vi "AlliGator All ROIs IRF Analysis.vi"(8 "error in (no error)":errorcluster, 11 "AlliGator Internal Variables DVR":refnum<data-value>) -> (0 "error out":errorcluster, 1 "# IRFs defined":i32, 2 "Message":string, 3 "AlliGator Internal Variables DVR":refnum<data-value>)   [LabVIEW 2021, in "AlliGator IRF.lvlib"]
doc: "Extracts the decays from all ROIs and stores them as IRFs for subsequent NLSF analysis."
uses:
  AlliGator IRF.lvlib
  Internal Variables/AlliGator Internal Variables v2.ctl
  <vilib>/vision/Image Controls.llb/IMAQ Image.ctl
  Internal Variables/AlliGator Gate Image Set.ctl
  Files/AlliGator FLI Dataset Type.ctl
  Files/AlliGator Data Series Type.ctl
  Dual-Channel Datasets/AlliGator Dataset Channel.ctl
  Settings/AlliGator Gate Arithmetic.ctl
  Source Image/AlliGator Displayed Image.ctl
  Image/Named ROI Description.ctl
  Phasor Graph/AlliGator Decay Metadata v3.ctl
  Decay Preprocessing/AlliGator Decay Background Subtraction Info.ctl
  Decay Preprocessing/AlliGator Baseline Subtraction Method.ctl
  Graphs/XY Graph/XY Graph Plot Shift Parameters.ctl
  Graphs/XY Graph/XY Graph Plot Shift Method.ctl
  Decay Preprocessing/AlliGator Decay Extrapolation Parameters.ctl
  Phasor/Calibration Phasor (m, phi).ctl
  Phasor/Phasor Reference Series.ctl
  Phasor/Phasor Calibration Map v2.ctl
  Phasor/Phasor (g, s).ctl
  Phasor Graph/AlliGator Raw Phasor Plot Data v5.ctl
  Phasor/Phasor Standard Deviation Options.ctl
  Phasor Plot/AlliGator Phasor Multi-Harmonic Data.ctl
  Phasor/Phasor Harmonic Data.ctl
  Decay Fit Parameter Map/AlliGator Decay Fit Options & Parameters v4.ctl
  Fits/IRF(X)PSED/Decay Fit Options v4.ctl
  Fits/Decay Convolution/Decay Model.ctl
  Fits/Residual Type.ctl
  Fits/IRF(X)PSED/Fit Weights Type v2.ctl
  Fits/Non-linear Fitting Method v2.ctl
  Fits/Fit Calculation Method.ctl
  Fits/Non-linear Fitting Algorithm.ctl
  Decay Fit/AlliGator Decay Fit Parameter Constraints 2.ctl
  Fits/IRF(X)PSED/Decay Fit Parameters In List.ctl
  Fits/IRF(X)PSED/MLE Baseline Offset Type.ctl
  Decay Preprocessing/AlliGator Decay Preprocessing Parameters.ctl
  Fits/IRF(X)PSED/Decay Fit Parameters & Derived Quantities List v2.ctl
  Fits/IRF(X)PSED/Decay Fit Result Constraint.ctl
  Decay Fit Parameter Map/AlliGator Parameter Maps Data.ctl
  Globals, Variables, Constants/AlliGator Variables List.ctl
  Rich Text Box/Text Format List.ctl
  Variant/Variant to Data/Variant to U16.vi
  <vilib>/Utility/error.llb/Error Cluster From Error Code.vi
  Globals, Variables, Constants/AlliGator Abort.vi
  <vilib>/ErrorRing/Error Ring.xnode
  Globals, Variables, Constants/AlliGator Globals, Variables & Constants.lvlib
  Image/Image.lvlib
  Decay Processing/AlliGator Decay Processing.lvlib
  Source Image/AlliGator Source Image.lvlib
  Strings/Strings.lvlib
  Time/Time.lvlib
  Decay Preprocessing/AlliGator Decay Preprocessing.lvlib
  Notebook/Notebook.lvlib
  GUI/GUI.lvlib
  Variant/Variant to Data/Variant to Data.lvlib
  Utilities/Utilities.lvlib
  Phasor/Phasor.lvlib
  Files/AlliGator Files.lvlib
  Internal Variables/AlliGator Internal Variables.lvlib
  Phasor Graph/AlliGator Phasor Graph.lvlib
  Graphs/XY Graph/XY Graph Add-Ons.lvlib
  Phasor Plot/AlliGator Phasor Plot.lvlib
  Fits/Fits.lvlib
  Decay Fit/AlliGator Decay Fit.lvlib
  Settings/AlliGator Settings.lvlib
  Dual-Channel Datasets/AlliGator Dual-Channel Datasets.lvlib
  Decay Fit Parameter Map/AlliGator Decay Fit Parameter Map.lvlib
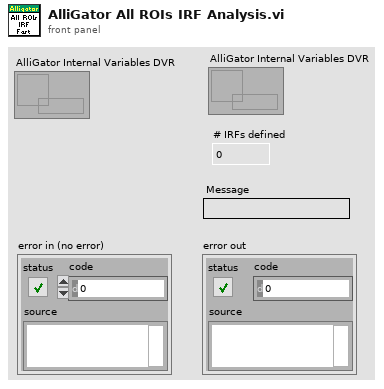
[diagram p1: front panel]
types:
  T1 = typedef "AlliGator Globals, Variables & Constants.lvlib/AlliGator Variables List.ctl" = enum16{"---- GUI ----", "GUI:Initialization Status", "GUI:State Indicators Refnum", "GUI:Original AlliGator Menu Items", "GUI:Current Action Loop State", "GUI:Script in progress", "GUI:Playback", "GUI:Loop Playback", "GUI:Search ROI Used", "GUI:Search ROI", "Decay Graph Max Legend Size", "Intensity Graph Max Legend Size", "Decay Statistics Graph Max Legend Size", "Phasor Graph Max Legend Size", "Phasor Ratio Graph Max Legend Size", "Lifetime Graph Max Legend Size", "---- Files ----", "Files:Export Dataset Frames as Individual Files", "Files:Show Batch Export Help Balloons", "Files:Frames in Dataset", "Files:ptu File Frame Start Indices", "Files:Current Frame in Dataset", "Files:Current Frame Timestamp", "Files:Dataset Loaded", "Files:Dataset Metadata", "Files:Dataset Channel", "Files:Dataset Data Description", "Files:Background Dataset Metadata", "Files:Background Dataset Channel", "Files:Background Dataset Data Description", "Files:Background File Subtraction", "Files:Background File Path", "Files:Background File Pile-up Correction", "Files:Background File Pixel Well Capacity", "Files:Background File Scaling Factor", "Files:Current Dataset Load Settings", "Files:Dataset Path", "Files:ICCD-specific Information", "Files:Macrotime Gate Separation", "------ Python Plugins ------", "Python Plugins:Information", "Python Plugins:Python Session", "Python Plugins:Valid Python Session?", "---- Source Image ----", "Source Image:ROIs", "Source Image:Current ROI", "Source Image:ROI Event Refnum", "X_Source Image:Display Range", "X_Source Image:Palette Information", "X_Source Image:Type of Displayed Image", "X_Time Gate Slider", "Source Image:Palette List", "Source Image:Scale", "Source Image:ROI Overlay Color", "Source Image:Overlay to Erase", "Source Image:Is Displayed Image Accumulated", "Source Image:White Light Image Modified", "Source Image:Mask Image Modified", "---- Image Profile Window ----", "Image Profile:Window Event Refnum", "Image Profile:IntensityType", "Image Profile:Intensity Average Type", "Image Profile:Intensity-weighted SDV", "Image Profile:Box Profile Type", "Image Profile:Window Open", "Image Profile:Plotted Fit Parameter", "------ Phasor Graph -------", "Phasor Graph:Show Line", "---- Phasor Plot ---", "Phasor Plot:Parameters Changed", "Phasor Plot:FLI Dataset Modified since last Calculation", "Phasor Harmonics Data", "Selected Phasor Harmonics", "Phasor Harmonic Manager Event Refnum", "Phasor Plot:ROIs", "Phasor Plot:Current ROI", "Phasor Plot:ROI Event Refnum", "Phasor Plot:Image Reference Points", "Phasor Plot:Computed", "Phasor Plot:Palette Information", "Phasor Plot:Palette List", "Phasor Plot:Phasor Ratio Palette Information", "Phasor Plot:Phasor Ratio Palette List", "Phasor Plot:Image Scale", "Phasor Plot:Image Overlay to Erase", "Phasor Plot:Image Elements to Update", "Phasor Plot:Current Calculation Parameters", "Phasor Plot:Current Calibration Options", "Phasor Plot:Reset Cumulated Phasor Plot", "Phasor Plot:Reference 1", "Phasor Plot:Lifetime Reference 1", "Phasor Plot:Reference 1 Frequency", "Phasor Plot:Reference 2", "Phasor Plot:Lifetime Reference 2", "Phasor Plot:Reference 2 Frequency", "---- Decay Analysis ----", "Number of Selected Decays to Fit", "LS Fit Results", "LAR Fit Results", "BS Fit Results", "Last Decay Max - Min", "Best Fit Parameters", "Best Fit Parameter Names", "Actual Size X", "Actual Size Y", "Binning X", "Binning Y", "Actual # Gates", "Dataset Number", "Gates to...", "Gates Skipped", "Gates to keep", "Gate Step", "Gate Separation", "Reversed Gates", "Pile-up Correction", "Pixel Well Capacity", "Background Subtracted", "Background Subtraction Method", "Background Definition Range", "Background File (deprecated)", "Number of Dataset Accumulated", "Array of Accumulated Dataset Paths", "Do Averaged Datasets", "Destination File Path", "Process Plot Target", "Use 1/D as Phasor Frequency", "---- Decay Fit Parameter Map -----", "Decay Fit Parameter Map:Palette Information", "Decay Fit Parameter Map:Palette List", "Decay Fit Parameter Map:X Resolution", "Decay Fit Parameter Map:Y Resolution", "Decay Fit Parameter Map:Use Decay Fit Result Constraints", "Decay Fit Parameter Map:Decay Fit Result Constraints", "Decay Fit Parameter Map:Decay Fit Result Constraints Applied", "---- Parameter Map ----", "Parameter Map:Palette Information", "Parameter Map:Palette List", "------- Local Decay Window ---------", "Local Decay Graph Window:Event Refnum", "Local Decay Graph Window:Use normalized IRF for convolution", "----- Miscellaneous ----", "Misc:Skippable Dialog Windows Status"}
  T2 = typedef "IMAQ Image.ctl" = refnum<image>
  T3 = typedef "Image.lvlib/Named ROI Description.ctl" = cluster{"ROI Descriptor":T4, "ROI Name":string, "Overlay Color":u32}
  T4 = typedef "ROI Descriptor" = cluster{"Global Rectangle":i32[], "Contours":cluster{"ID":enum32{"External", "Internal"}, "Type":u32, "Coordinates":i32[]}[]}
  T5 = typedef "Notebook.lvlib/Text Format List.ctl" = enum16{"Message", "Result", "Error", "Setting", "Verbose", "Warning"}
  T6 = typedef "AlliGator Internal Variables.lvlib/AlliGator Internal Variables v2.ctl" = cluster{"----------------------------- Images -----------------------------":u8, "Displayed Image":T2, "White Light Image":T2, "Mask Image":T2, "ROI Mask Image":T2, "Current Dataset Images 1":T7, "Background Dataset Images 1":T7, "Current Dataset Images 2":T7, "Background Dataset Images 2":T7, "Current Dataset Arithmetic Images":T7, "Accumulated Dataset Images 1":T7, "Accumulated Dataset Images 2":T7, "Accumulated Dataset Arithmetic Images":T7, "----------------------------- File Paths -----------------------------":u8, "Phasor Plot Image":T2, "Decay Fit Parameter Map Image":T2, "Parameter Map Image":T2, "Single Data Point Path":path, "White Light Image Path":path, "Mask Image Path":path, "Time-Series Folder":path, "[Time-Series Paths]":path[], "----------------------------- FLI Dataset -----------------------------":u8, "Current Dataset":i32, "Single Dataset Type":T8, "Current Folder":string, "AlliGator Data Series Type":T9, "# Datasets":i32, "Dual-Channel Dataset":bool, "Selected Channel Name":string, "Dataset Channel":T10, "Channel Arithmetic":T11, "Dual-Channel Background Dataset":bool, "Background Channel":T10, "Dual-Channel Accumulated Dataset":bool, "Start Time":dbl, "[Time-Series Timestamps]":dbl[], "[Intensity Corrections]":dbl[], "Time Series Script":bool, "Type of Displayed Image":T12, "Gate Image Slide":u16, "# Gates":i32, "ROIs":T3[], "----------------------------- Decays -----------------------------":u8, "ROI Decay":cluster{"t Array":dbl[], "I Array":dbl[]}, "Valid Decay":bool, "Decay  Metadata":T13, "Reference Decay Plot Name":string, "Reference Decay":cluster{"t Array":dbl[], "I Array":dbl[]}, "Decay Shift Plot":cluster{"Time Stamps":dbl[], "Decay Shifts":dbl[]}, "[Decays Max Values]":sgl[], "[Decays Min Values]":sgl[], "----------------------------- Calibration -----------------------------":u8, "Calibration Phasor":T19, "Calibration Phasor Series":T20, "Phasor Calibration Map":T21, "Calibration Map MD5 Digest":string, "----------------------------- Phasor Graph -----------------------------":u8, "Last Raw Phasor":T22, "Last Calibrated Phasor":T22, "Last Calibrated Phasor SDV":T22, "Phasor Graph:Phasor Plot":cluster{"g Array":dbl[], "s Array":dbl[]}, "Phasor Graph:Phasor SDV Plot":cluster{"g Array":dbl[], "s Array":dbl[]}, "[Phasor Graph:Raw Phasor Plots]":T23[], "Phasor Plot locked to Ref 1":i32, "[Phasor Plot(s) locked to Ref 1]":i32[], "[Phasor Plot(s) locked to Ref 2]":i32[], "[Pixel Phasors]":T22[], "----------------------------- Phasor Plot -----------------------------":u8, "[[Sum Image]]":dbl[][], "[[CSG Phasors]]":csg[][], "[[Valid Pixel?]]":bool[][], "[[Phasor Ratios]]":dbl[][], "[[Average Lifetimes]]":dbl[][], "Amplitude Weighted Average Lifetime":bool, "I/m/phi Dataset":cluster{"I/m/phi Dataset?":bool, "Base Frequency":dbl[unit], "Harmonic Orders":u8[]}, "Multi Phasor Plot Data":T25, "----------------------------- Decay Fit Parameter Map -----------------------------":u8, "Decay Fit Options & Parameters":T27, "Fit Options: Decay Preprocessing Parameters":T38, "Fit Options: Reference Decay":cluster{"t Array":dbl[], "I Array":dbl[]}, "Is Full Image Parameters Map":bool, "Is Single-Pixels Parameters Map":bool, "NLSF Parameters Map X Resolution":i32, "NLSF Parameters Map Y Resolution":i32, "[Single Decay Fit Parameters]":dbl[], "Fit Model":T29, "[[Multiple Decays Fit Parameters]]":dbl[][], "[[Multiple Decays Fit Parameter SDVs]]":dbl[][], "[[IRFs]]":dbl[][], "[ROI Descriptors]":T4[], "IRF Array Time Axis":dbl[], "Decay Array Time Axis":dbl[], "[Decay Fit Parameter Names]":T39[], "[Decay Sum]":dbl[], "Array of Decay Fit Result Constraints":T40[], "Selected ROIs Array":bool[], "----------------------------- Parameter Maps -----------------------------":u8, "[Map Set Names]":string[], "[Parameter Maps]":T41[], "[[User-defined Quantities]]":dbl[][], "User-defined Quantity":string}
  T7 = typedef "AlliGator Internal Variables.lvlib/AlliGator Gate Image Set.ctl" = cluster{"SGL Gate Images":T2[], "SGL Sum Image":T2, "SGL Max Image":T2, "SGL Min Image":T2}
  T8 = typedef "AlliGator Files.lvlib/AlliGator FLI Dataset Type.ctl" = enum16{"HDF5 FLI Dataset", "Gate Image Folder", ".sdt FLI Dataset (Becker & Hickl)", ".ptu FLI Dataset (PicoQuant)", "SS1 FLI Dataset", "SS2 FLI Dataset", "I/m/phi Dataset", ".bin FLI Dataset (PicoQuant Binned)", ".bin FLI Dataset (Piccolo Binned)", ".mat FLI Dataset"}
  T9 = typedef "AlliGator Files.lvlib/AlliGator Data Series Type.ctl" = enum16{"Not a Supported Series", "Gate Images Folder Series", "SwissSPAD 2 Dataset Series", "B&H FLI Dataset Series", "PicoQuant PTU FLI Dataset Series", "PicoQuant BIN FLI Dataset Series", "Piccolo hist BIN FLI Dataset Series", "HDF5 FLI Dataset Series"}
  T10 = typedef "AlliGator Dual-Channel Datasets.lvlib/AlliGator Dataset Channel.ctl" = enum16{"G2", "INT"}
  T11 = typedef "AlliGator Settings.lvlib/AlliGator Gate Arithmetic.ctl" = enum16{"None", "INT-G2", "G2/INT*<INT>", "(1 - G2/INT)*<INT>"}
  T12 = typedef "AlliGator Source Image.lvlib/AlliGator Displayed Image.ctl" = enum16{"Single Gate", "Sum of All Gates", "Max of All Gates", "Min of All Gates", "-", "White Ligth Image", "Mask Image"}
  T13 = typedef "AlliGator Phasor Graph.lvlib/AlliGator Decay Metadata v3.ctl" = cluster{"ROI Descriptor":T4, "ROI Center":cluster{"X":i32, "Y":i32}, "Decay Background Subtraction Info":T14, "Decay Reverted":bool, "Decay Smoothened":bool, "Decay Straightened":bool, "Fitted Tau (Decay Straightening)":dbl, "Decay Shift Parameters":T16, "Decay Shifted":bool, "Decay Extrapolated":bool, "Decay Extrapolation Parameters":T18, "Decay Normalized":bool, "Fold Decay":bool, "# Folds":u32}
  T14 = typedef "AlliGator Decay Preprocessing.lvlib/AlliGator Decay Background Subtraction Info.ctl" = cluster{"Laser Period":dbl[unit], "Gate Duration":dbl[unit], "Baseline Subtraction Method":T15, "Background Definition Range":cluster{"Min Gate":dbl[unit], "Max Gate":dbl[unit]}, "Total Intensity w/o Bkgd Subtraction":dbl, "Bkgd-subtracted Intensity (exp)":dbl, "# Data Points":i32, "Background/Gate":dbl, "Fitted Lifetime":dbl[unit], "Bkgd-subtracted Intensity (theo)":dbl}
  T15 = typedef "AlliGator Decay Preprocessing.lvlib/AlliGator Baseline Subtraction Method.ctl" = enum16{"Mean", "Min", "Square Gated Single-Exponential", "File", "Constant"}
  T16 = typedef "XY Graph Add-Ons.lvlib/XY Graph Plot Shift Parameters.ctl" = cluster{"Type":T17, "Shift":dbl[unit], "Threshold":dbl, "Rotate":bool}
  T17 = typedef "XY Graph Add-Ons.lvlib/XY Graph Plot Shift Method.ctl" = enum16{"Default", "CFD", "Threshold", "Cross-Correlation"}
  T18 = typedef "AlliGator Decay Preprocessing.lvlib/AlliGator Decay Extrapolation Parameters.ctl" = cluster{"Additional Points":u32, "Head Fraction":dbl, "Fitted Tau":dbl, "Use Periodicity":bool, "Use Cursors":bool, "Tail Fraction":dbl}
  T19 = typedef "Phasor.lvlib/Calibration Phasor (m, phi).ctl" = cluster{"m":dbl, "phi":dbl, "Phasor Frequency":dbl[unit], "Reference Lifetime":dbl[unit]}
  T20 = typedef "Phasor.lvlib/Phasor Reference Series.ctl" = cluster{"m Array":dbl[], "phi Array":dbl[], "Phasor Frequency":dbl[unit], "Calibration Lifetime":dbl[unit]}
  T21 = typedef "Phasor.lvlib/Phasor Calibration Map v2.ctl" = cluster{"Phasor Frequency":dbl[unit], "Calibration Lifetime":dbl[unit], "ROI Centers":cluster{"X":i32, "Y":i32}[], "ROI Descriptors":T4[], "Map Resolution X":i32, "Map Resolution Y":i32, "z Array":cdb[]}
  T22 = typedef "Phasor.lvlib/Phasor (g, s).ctl" = cluster{"g":dbl, "s":dbl}
  T23 = typedef "AlliGator Phasor Graph.lvlib/AlliGator Raw Phasor Plot Data v5.ctl" = cluster{"Phasor Plot Name":string, "Raw Phasor Plot":T22[], "Phasor Frequency":dbl[unit], "[Decay Metadata]":T13[], "Raw Phasor Plot SDV":T22[], "Phasor SDV Options":T24, "[Calibration Phasor]":T19[], "Intensity Array":dbl[]}
  T24 = typedef "Phasor.lvlib/Phasor Standard Deviation Options.ctl" = cluster{"Compute Estimated SDV":bool, "# Replicas":u32, "Use Estimated Average Phasor":bool}
  T25 = typedef "AlliGator Phasor Plot.lvlib/AlliGator Phasor Multi-Harmonic Data.ctl" = cluster{"Base Frequency":dbl[unit], "# Harmonics":u8, "Harmonic Orders":u8[], "Phasor Plot Settings Checksum":u64, "Phasor Harmonic Data Array":T26[]}
  T26 = typedef "Phasor.lvlib/Phasor Harmonic Data.ctl" = cluster{"Phasor Harmonic Name":string, "Phasor Plot Settings Checksum":u64, "Phasor Frequency":dbl[unit], "Base Frequency":dbl[unit], "Harmonic Order":u8, "Phasor Plot Parameters":string, "Phasor Array [[CSG]]":csg[][], "Dataset File Path":path}
  T27 = typedef "AlliGator Decay Fit Parameter Map.lvlib/AlliGator Decay Fit Options & Parameters v4.ctl" = cluster{"SYNC Period":dbl[unit], "Fit Options":T28, "Fit Parameter Constraints":T35[], "MLE Baseline Offset":dbl, "MLE Baseline Offset Type":T37}
  T28 = typedef "Fits.lvlib/Decay Fit Options v4.ctl" = cluster{"Show Fit Residuals":bool, "Fit Model":T29, "Residual Type":T30, "Max Decay Percentile":dbl, "Min Decay Percentile":dbl, "Show Full Decay":bool, "Weights":T31, "Fitting Method":T32, "Compute Parameter Uncertainties":bool, "Periodic Boundaries":bool, "Model Calculation":T33, "Period":dbl[unit], "Termination Criteria":cluster{"Max Iterations":i32, "Max Function Calls":i32, "Max Time":dbl[unit], "Function Tolerance":dbl, "Parameter Tolerance":dbl, "Gradient Tolerance":dbl, "Min Lambda":dbl, "Max Lambda":dbl, "Initial Tick Count":u32}, "Offset Resolution":dbl[unit], "Use Local IRF":bool, "Fitting Algorithm":T34, "Show Confidence Interval ":bool, "Confidence Level":dbl}
  T29 = typedef "Fits.lvlib/Decay Model.ctl" = enum16{"1-Exponential", "2-Exponentials"}
  T30 = typedef "Fits.lvlib/Residual Type.ctl" = enum16{"Standard", "Normalized", "Reduced"}
  T31 = typedef "Fits.lvlib/Fit Weights Type v2.ctl" = enum16{"Unweighted", "1/Variance (Neyman)", "1/Variance (Pearson)", "Best of All"}
  T32 = typedef "Fits.lvlib/Non-linear Fitting Method v2.ctl" = enum16{"Least Square", "Least Absolute Residual", "Bisquare", "MLE", "-", "Best of All"}
  T33 = typedef "Fits.lvlib/Fit Calculation Method.ctl" = enum16{"Simulation", "Convolution", "Integration"}
  T34 = typedef "Fits.lvlib/Non-linear Fitting Algorithm.ctl" = enum16{"Levenberg-Marquardt", "Trust-Region Dogleg"}
  T35 = typedef "AlliGator Decay Fit.lvlib/AlliGator Decay Fit Parameter Constraints 2.ctl" = cluster{"Fit Parameter":T36, "Min Value":dbl, "Max Value":dbl, "Global":bool, "Used":bool}
  T36 = typedef "Fits.lvlib/Decay Fit Parameters In List.ctl" = enum16{"Offset", "Baseline", "A_1", "tau_1", "A_2", "tau_2"}
  T37 = typedef "Fits.lvlib/MLE Baseline Offset Type.ctl" = enum32{"Absolute", "Percentage"}
  T38 = typedef "AlliGator Decay Preprocessing.lvlib/AlliGator Decay Preprocessing Parameters.ctl" = cluster{"Background Subtraction":bool, "Straighten Decay":bool, "Reverse Gates":bool, "1-Normalized Decay":bool, "Smoothen Decay":bool, "Smoothing Parameter":dbl, "Shift Decay":bool, "Decay Shift Parameters":T16, "Extrapolate Decay":bool, "Additional Points":u32, "Head Fraction":dbl, "Pixel-Normalize Decay":bool, "Use Periodicity":bool, "Use Cursors":bool, "Tail Fraction":dbl, "Use Decay Pre-Processing":bool, "Fold Decay":bool, "# Folds":u32, "[0-1]-Normalized Decay":bool}
  T39 = typedef "Fits.lvlib/Decay Fit Parameters & Derived Quantities List v2.ctl" = enum16{"Offset", "Baseline", "A_1", "tau_1", "A_2", "tau_2", "<tau>_a", "f1_a", "f2_a", "<tau>_i", "f1_i", "f2_i", "-", "R^2", "Chi^2"}
  T40 = typedef "Fits.lvlib/Decay Fit Result Constraint.ctl" = cluster{"Fit Parameter":enum16{"Offset", "Baseline", "A_1", "tau_1", "A_2", "tau_2", "<tau>_a", "f1_a", "f2_a", "<tau>_i", "f1_i", "f2_i", "-", "R^2", "Chi^2", "Max Relative Residual", "<Residual ACF>", "Residual ACF SDV", "tau_2/tau_1"}, "Min Value":dbl, "Max Value":dbl, "Use Constraint":bool}
  T41 = typedef "AlliGator Decay Fit Parameter Map.lvlib/AlliGator Parameter Maps Data.ctl" = cluster{"Map Set Name":string, "[Parameter Names]":string[], "[[Parameters]]":dbl[][], "[[Parameter SDVs]]":dbl[][], "Decay Array Time Axis":dbl[], "[[IRFs]]":dbl[][], "IRF Array Time Axis":dbl[], "X Resolution":i32, "Y Resolution":i32, "Intensity Array":dbl[]}
  T42 = typedef "AlliGator Settings.lvlib/AlliGator Pixel Counts Constraints.ctl" = cluster{"High Count Pixels Rejection Options":T43, "Low Count Pixels Rejection Options":T44}
  T43 = typedef "AlliGator Settings.lvlib/AlliGator High Count Pixels Rejection Options.ctl" = cluster{"Background High Threshold Factor":dbl, "Fixed High Background Threshold":dbl, "Reject High Count Pixels":bool, "High Percentile":dbl}
  T44 = typedef "AlliGator Settings.lvlib/AlliGator Low Count Pixels Rejection Options.ctl" = cluster{"Background Low Threshold Factor":dbl, "Fixed Low Background Threshold":dbl, "Reject Low Count Pixels":bool, "Low Percentile":dbl}
  T45 = cluster{"Decay Peak Constraint":bool, "Min":dbl, "Max":dbl}
  T46 = typedef "Rich Text Box.lvlib/Text Formatting.ctl" = cluster{"Font":string, "Text Color":T47, "Background Color":T47, "Style":T48, "Font Size":dbl, "Alignment":T49}
  T47 = typedef "Rich Text Box.lvlib/Text Colors.ctl" = enum16{"Unchanged", "Black", "Blue", "Cyan", "Maroon", "Gray", "Violet", "Green", "Light Green", "Orange", "Yellow", "Magenta", "Red", "White"}
  T48 = typedef "Rich Text Box.lvlib/Text Style.ctl" = enum16{"Regular", "Bold", "Italic", "Underline", "Strikeout"}
  T49 = typedef "Rich Text Box.lvlib/Text Alignment.ctl" = enum16{"Left", "Right", "Center"}
  T50 = cluster{"t Axis":dbl[], "ROI Intensity Array":dbl[]}
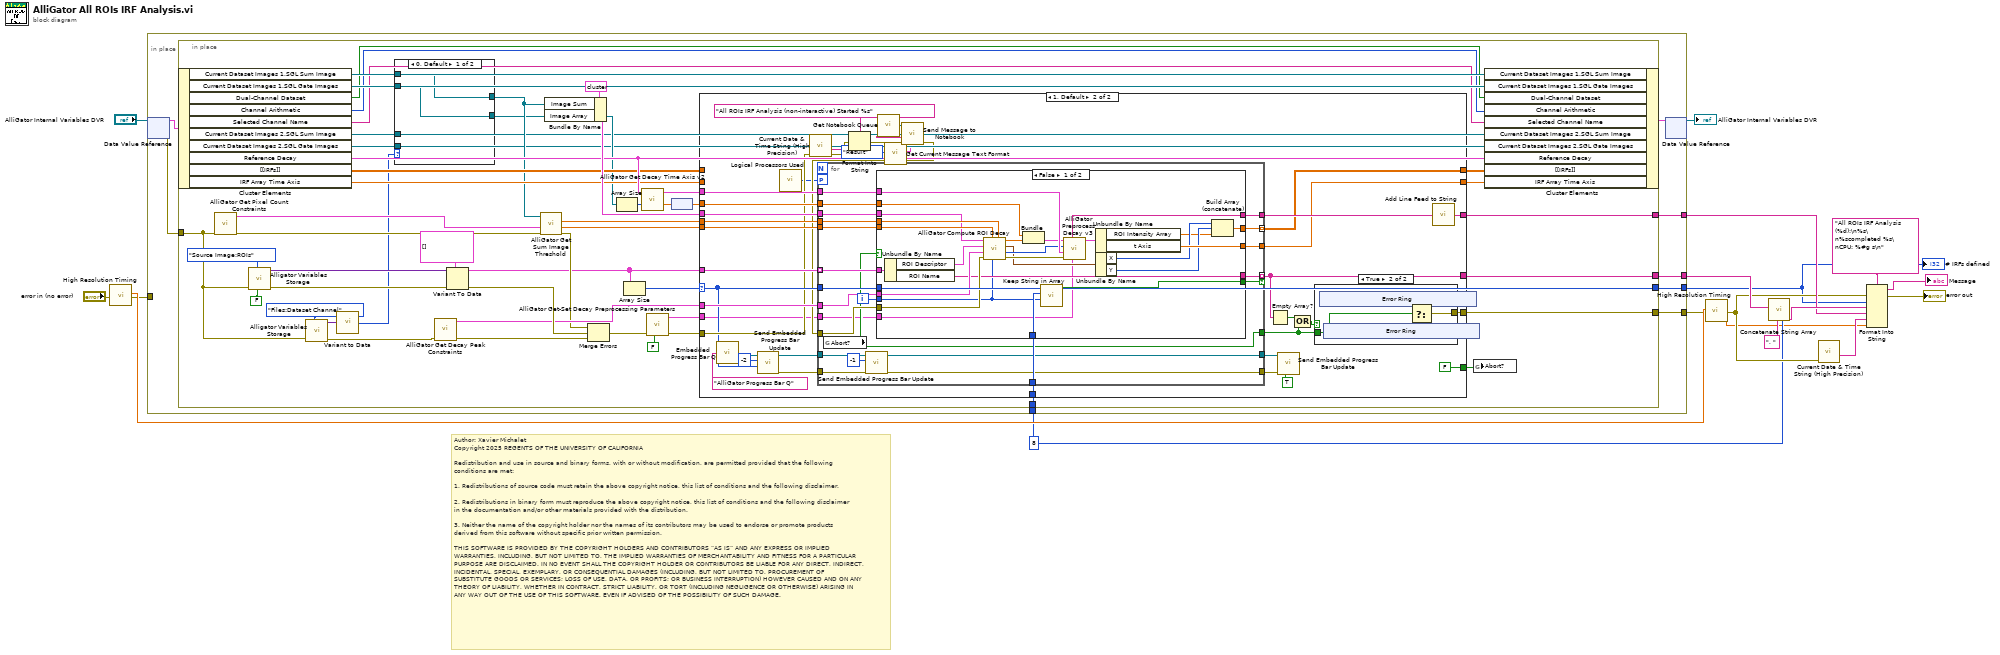
[diagram p0: block diagram]
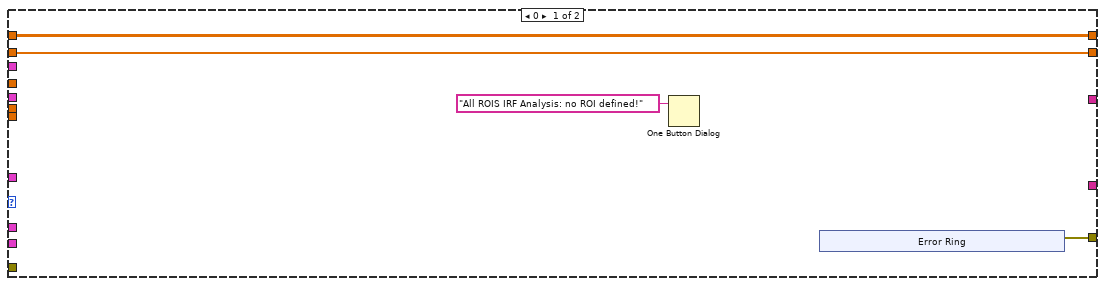
[diagram p3: hidden frame]
diagram:
  w6 = 8 ("Max Number of Elements (None: -1)")
  # "Author: Xavier Michalet\nCopyright 2025 REGENTS OF THE UNIVERSITY OF CALIFORNIA\n\nRedistribution and use in source and binary forms, with or without modification, are permitted provided that the following conditions are met:\n\n1. Redistributions of source code must retain the above copyright notice, this list of conditions and the following disclaimer.\n\n2. Redistributions in binary form must reproduce the above copyright notice, this list of conditions and the following disclaimer in the documentation and/or other materials provided with the distribution.\n\n3. Neither the name of the copyright holder nor the names of its contributors may be used to endorse or promote products derived from this software without specific prior written permission.\n\nTHIS SOFTWARE IS PROVIDED BY THE COPYRIGHT HOLDERS AND CONTRIBUTORS “AS IS” AND ANY EXPRESS OR IMPLIED WARRANTIES, INCLUDING, BUT NOT LIMITED TO, THE IMPLIED WARRANTIES OF MERCHANTABILITY AND FITNESS FOR A PARTICULAR PURPOSE ARE DISCLAIMED. IN NO EVENT SHALL THE COPYRIGHT HOLDER OR CONTRIBUTORS BE LIABLE FOR ANY DIRECT, INDIRECT, INCIDENTAL, SPECIAL, EXEMPLARY, OR CONSEQUENTIAL DAMAGES (INCLUDING, BUT NOT LIMITED TO, PROCUREMENT OF SUBSTITUTE GOODS OR SERVICES; LOSS OF USE, DATA, OR PROFITS; OR BUSINESS INTERRUPTION) HOWEVER CAUSED AND ON ANY THEORY OF LIABILITY, WHETHER IN CONTRACT, STRICT LIABILITY, OR TORT (INCLUDING NEGLIGENCE OR OTHERWISE) ARISING IN ANY WAY OUT OF THE USE OF THIS SOFTWARE, EVEN IF ADVISED OF THE POSSIBILITY OF SUCH DAMAGE."
  n1 = call "High Resolution Timing.vi"("Error In"="error in (no error)") -> ("elapsed (relative) seconds"=w13:dbl, "Error Out"=w10:errorcluster)  [unwired: 16 in, 1 out]
  n2 = in-place {
    in-place-border: [w24] -> w7
    in-place-border: [w23] -> w11
    in-place-border: w10 -> [_]
    in-place-border: [w21] -> w9
    in-place-border: [w20] -> w5
    in-place-border: w6 -> [w19]
    n3 = in-place-dvr #1("AlliGator Internal Variables DVR") -> (w26:T6, w22:errorcluster)
    n4 = in-place {
      in-place-border: w22 -> [w30]
      in-place-border: [w58] -> w24
      in-place-border: [w49] -> w23
      in-place-border: [w57] -> w21
      in-place-border: [w51] -> w20
      in-place-border: w19 -> [w50]
      n5 = in-place-cluster #2(w26) -> ("Current Dataset Images 1.SGL Sum Image"=w39:T2, "Current Dataset Images 1.SGL Gate Images"=w38:T2[], "Dual-Channel Dataset"=w33:bool, "Channel Arithmetic"=w34:T11, "Selected Channel Name"=w35:string, "Current Dataset Images 2.SGL Sum Image"=w37:T2, "Current Dataset Images 2.SGL Gate Images"=w36:T2[], "Reference Decay"=w59:cluster{"t Array":dbl[], "I Array":dbl[]}, "[[IRFs]]"=w46:dbl[][], "IRF Array Time Axis"=w45:dbl[])
      n6 = call "AlliGator Get Pixel Count Constraints.vi"("error in (no error)"=w30) -> ("error out"=w68:errorcluster, "Pixel Count Constraints"=w69:T42)  [unwired: 9 in]
      n7 = call "Alligator Variables Storage.vi"("Get(F)/Set"=FALSE, "AlliGator Variable"=AlliGator_Variables_List."Source Image:ROIs" ("Alligator Variable"), "Error In"=w30) -> ("Error Out"=w72:errorcluster, "Data out"=w73:variant)  [unwired: 6 in, 1 out]
      n8 = call "Alligator Variables Storage.vi"("AlliGator Variable"=AlliGator_Variables_List."Files:Dataset Channel" ("Alligator Variable"), "Error In"=w30) -> ("Error Out"=w29:errorcluster, "Data out"=w31:variant)  [unwired: 7 in, 1 out]
      n9 = call-poly "Variant to Data.vi"("Variant"=w31) -> ("U16 Value"=w28:u16)  [unwired: 8 in]
      n10 = case shown="0, Default" w28 {
        tunnel: [w76 w78] -> w41
        tunnel: w37 -> [_ w78]
        tunnel: [w75 w77] -> w40
        tunnel: w36 -> [_ w77]
        tunnel: w39 -> [w76 _]
        tunnel: w38 -> [w75 _]
        frame 0, Default {
        }
        frame 1 {
        }
      }
      n11 = call "AlliGator Get Decay Peak Constraints.vi"("error in (no error)"=w29) -> ("Error Out"=w64:errorcluster, "Decay Peak Constraints"=w63:T45)  [unwired: 9 in]
      n12 = Variant To Data(error in=w72, type=T3[] [] ("Stored ROIs in"), Variant=w73) -> (data=w52:T3[], error out=w67:errorcluster)
      n13 = call "AlliGator Get Sum Image Threshold.vi"("error in (no error)"=w68, "Pixel Counts Constraints"=w69, "Image in"=w41) -> ("error out"=w56:errorcluster, "Pixel Threshold Low"=w65:sgl, "Pixel Threshold High"=w66:sgl)  [unwired: 2 in, 4 out]
      n14 = Bundle By Name(cluster=cluster{"Image Sum":T2, "Image Array":T2[]} {"Image Sum"=refnum, "Image Array"=[]} ("Images"), "Image Sum"=w41, "Image Array"=w40) -> (w62:cluster{"Image Sum":T2, "Image Array":T2[]})
      n15 = Merge Errors(w56, w67, w64) -> (w48:errorcluster)
      n16 = Array Size(array=w40) -> (size(s)=w61:i32)
      n17 = Array Size(array=w52) -> (size(s)=w51:i32)
      n18 = call "AlliGator Get Decay Time Axis v2.vi"("Number of Gates"=w61) -> ("t Array"=w60:dbl[unit][])  [unwired: 14 in]
      n19 = call "AlliGator Get-Set Decay Preprocessing Parameters.vi"("Get (F)/Set"=FALSE, "Error In"=w48) -> ("Error Out"=w47:errorcluster, "Decay Preprocessing Parameters out"=w43:T38)  [unwired: 8 in]
      n20 = node(w60) -> (w55:dbl[])
      n21 = case shown="1, Default" w51 {
        selector: w51 -> [_ w96]
        tunnel: w66 -> [_ w125]
        tunnel: w65 -> [_ w124]
        tunnel: w63 -> [_ w123]
        tunnel: w62 -> [_ w122]
        tunnel: w59 -> [_ w121]
        tunnel: [w80 w120] -> w58
        tunnel: [_ w116] -> w57
        tunnel: w55 -> [_ w115]
        tunnel: [w81 w113] -> w54
        tunnel: [w82 w112] -> w53
        tunnel: w52 -> [_ w111]
        tunnel: w50 -> [_ w110]
        tunnel: [_ w109] -> w49
        tunnel: w47 -> [_ w102]
        tunnel: w46 -> [w82 _]
        tunnel: w45 -> [w81 _]
        tunnel: w43 -> [_ w91]
        tunnel: [_ FALSE ("Abort?")] -> w27
        frame 0 {
          n22 = One Button Dialog(message="All ROIS IRF Analysis: no ROI defined!") -> ()  [unwired: 1 in, 1 out]
          n23 = xnode "Error Ring"() -> ("error out"=w80:errorcluster)
        }
        frame 1, Default {
          n24 = call "Embedded Progress Bar Q.vi"("Progress Bar Queue Name"="AlliGator Progress Bar Q") -> ("Progress Bar Queue"=w99:refnum<queue>)  [unwired: 6 in]
          n25 = call "Send Embedded Progress Bar Update.vi"("Max Iterations N"=w96, "Current Iteration i (i or -1: standard or || iteration; 0 or -2: first standard or || iteration)"=-2 ("Current Iteration i (-1: || iteration, -2: first || iteration)"), "Progress Bar Queue in"=w99) -> ("Error Out"=w95:errorcluster, "Progress Bar Queue out"=w97:refnum<queue>)  [unwired: 7 in]
          n26 = call "Logical Processors Used.vi"() -> ("# Logical Processor Used"=w89:i32)  [unwired: 6 in]
          n27 = call "Current Date & Time String (High Precision).vi"("Error In"=w102) -> ("Error Out"=w104:errorcluster, "on <Date> at <Time>"=w90:string)  [unwired: 7 in, 2 out]
          n28 = Format Into String(format string="All ROIs IRF Analysis (non-interactive) Started %s", error in=w104, w90) -> (resulting string=w101:string, error out=w106:errorcluster)  [unwired: 1 in]
          n29 = call "Get Notebook Queue.vi"() -> ("Notebook Queue"=w105:refnum<queue>)  [unwired: 9 in]
          n30 = call "Get Current Message Text Format.vi"("Text Format"=Text_Format_List."Result") -> ("Message Formatting"=w107:T46)  [unwired: 8 in, 1 out]
          n31 = call "Send Message to Notebook.vi"("Text Formatting"=w107, "Error In"=w106, "Text"=w101, "Notebook Queue"=w105) -> ("Error Out"=w103:errorcluster)  [unwired: 4 in, 1 out]
          n32 = for {
            tunnel: w111 -> [w160] mode=indexing
            tunnel: w125 -> [w159]
            tunnel: w124 -> [w158]
            tunnel: w122 -> [w157]
            tunnel: w123 -> [w156]
            tunnel: [w144] -> w114
            tunnel: w115 -> [w152]
            tunnel: w121 -> [w153]
            tunnel: [w154] -> w109 mode=indexing if=w148
            tunnel: w103 -> [w155]
            tunnel: [w151] -> w117
            tunnel: [w150] -> w113
            tunnel: [w149] -> w112 mode=indexing
            tunnel: w96 -> [w146]
            tunnel: w110 -> [w145]
            tunnel: w97 -> [w142]
            tunnel: w95 -> [w141]
            tunnel: [w140] -> w94
            tunnel: [w139] -> w93
            tunnel: w91 -> [w138]
            workers-P: w89 -> [_]
            i -> [w147]
            n33 = global read "AlliGator Abort.vi" "Abort?"() -> (w144:bool)
            n34 = call "Send Embedded Progress Bar Update.vi"("Error In"=w141, "Current Iteration i (i or -1: standard or || iteration; 0 or -2: first standard or || iteration)"=-1 ("Current Iteration i (-1: || iteration, -2: first || iteration)"), "Progress Bar Queue in"=w142) -> ("Error Out"=w139:errorcluster, "Progress Bar Queue out"=w140:refnum<queue>)  [unwired: 7 in]
            n35 = case shown="False" w144 {
              tunnel: w160 -> [w187 _]
              tunnel: w159 -> [w186 _]
              tunnel: w158 -> [w185 _]
              tunnel: w157 -> [w184 _]
              tunnel: w156 -> [w183 _]
              tunnel: w155 -> [w182 _]
              tunnel: [w181 _] -> w154
              tunnel: w153 -> [w179 _]
              tunnel: w152 -> [w177 _]
              tunnel: [w174 _] -> w151
              tunnel: [w170 _] -> w150
              tunnel: [w166 _] -> w149
              tunnel: [w165 _] -> w148
              tunnel: w147 -> [w161 _]
              tunnel: w146 -> [w164 _]
              tunnel: w145 -> [w163 _]
              tunnel: w138 -> [w162 _]
              frame False {
                n36 = Unbundle By Name(w187) -> ("ROI Descriptor"=w180:T4, "ROI Name"=w181:string)
                n37 = call "AlliGator Compute ROI Decay.vi"("Pixel Threshold High"=w186, "Loop ID"=w161, "Pixel Threshold Low"=w185, "error in (no error)"=w182, "Decay Peak  Constraints"=w183, "ROI Descriptor"=w180, "Images"=w184) -> ("error out"=w178:errorcluster, "# Valid Pixels"=w173:i32, "ROI Center"=w171:cluster{"X":i32, "Y":i32}, "Decay Points"=w176:dbl[])  [unwired: 1 out]
                n38 = Bundle(w177, "Decay Points"=w176) -> (w175:cluster{dbl[], "Decay Points":dbl[]})  [unwired: 1 in]
                n39 = call "Keep String in Array.vi"("Current Index"=w161, "Max Number of Strings (8)"=w163, "Number of Elements"=w164) -> ("Keep String"=w165:bool)  [unwired: 8 in]
                n40 = call "AlliGator Preprocess Decay v3.vi"("Decay Preprocessing Parameters"=w162, "Error In"=w178, "Time-Gated Reference Decay"=w179, "# Pixels"=w173, "Decay (in)"=w175) -> ("Decay (out)"=w172:T50, "Message"=w174:string)  [unwired: 3 in, 2 out]
                n41 = Unbundle By Name(w172) -> ("ROI Intensity Array"=w167:dbl[], "t Axis"=w170:dbl[])
                n42 = Unbundle By Name(w171) -> ("X"=w169:i32, "Y"=w168:i32)
                n43 = Build Array (concatenate)(w169, w168, w167) -> (w166:dbl[])
              }
              frame True {
              }
            }
          }
          n44 = Empty Array?(array=w109) -> (empty?=w118:bool)
          n45 = call "Send Embedded Progress Bar Update.vi"("Stop Progress Bar (F)"=TRUE, "Error In"=w93, "Progress Bar Queue in"=w94) -> ()  [unwired: 7 in, 2 out]
          n46 = Compound Arithmetic op=OR(w118, w114) -> (w119:bool)
          n47 = case shown="True" w119 {
            tunnel: [_ w127] -> w120
            tunnel: w114 -> [_ w129]
            frame False {
            }
            frame True {
              n48 = xnode "Error Ring"() -> ("error out"=w128:errorcluster)
              n49 = xnode "Error Ring"() -> ("error out"=w126:errorcluster)
              n50 = Select(t=w128, s=w129, f=w126) -> (s? t:f=w127:errorcluster)
            }
          }
          n51 = call "Add Line Feed to String.vi"("String"=w117) -> ("String\\n"=w116:string)  [unwired: 8 in]
        }
      }
      n52 = global write "AlliGator Abort.vi" "Abort?"(w27) -> ()
      n53 = in-place-cluster #2("Current Dataset Images 1.SGL Sum Image"=w39, "Current Dataset Images 1.SGL Gate Images"=w38, "Dual-Channel Dataset"=w33, "Channel Arithmetic"=w34, "Selected Channel Name"=w35, "Current Dataset Images 2.SGL Sum Image"=w37, "Current Dataset Images 2.SGL Gate Images"=w36, "Reference Decay"=w59, "[[IRFs]]"=w53, "IRF Array Time Axis"=w54) -> (w25:T6)
    }
    n54 = in-place-dvr #1(w25) -> (→"AlliGator Internal Variables DVR":refnum<data-value>)  [unwired: 1 out]
  }
  "# IRFs defined" <- w5
  n55 = call "High Resolution Timing.vi"("relative seconds (NaN)"=w13, "Error In"=w7) -> ("elapsed (relative) seconds"=w2:dbl, "Error Out"=w8:errorcluster)  [unwired: 15 in, 1 out]
  n56 = call "Concatenate String Array.vi"("Max Number of Elements (None: -1)"=w6, "Separator (TAB)"=", ", "String Array"=w11) -> ("Formatted String"=w12:string)  [unwired: 8 in]
  n57 = call "Current Date & Time String (High Precision).vi"("Error In"=w8) -> ("on <Date> at <Time>"=w3:string)  [unwired: 7 in, 3 out]
  n58 = Format Into String(format string="All ROIs IRF Analysis (%d):\n%s\n%scompleted %s\nCPU: %#g s\n", error in=w8, w5, w12, w9, w3, w2) -> (resulting string=→"Message":string, error out=→"error out":errorcluster)  [unwired: 1 in]
